vi "Build Swept Freq Vectors.vi"(5 "Low or High (T=Low)":bool=TRUE, 6 "Freq. Increment MHz":dbl=0.001 min=0.001, 7 "Base Order (0)":u8, 8 "Carrier 2":cluster{"Low Freq":dbl, "High Freq":dbl} {"Low Freq" format="%.2f"; "High Freq" format="%.2f"}, 9 "Carrier 1":cluster{"Low Freq":dbl, "High Freq":dbl} {"Low Freq" format="%.2f"; "High Freq" format="%.2f"}, 10 "Rx High Freq":dbl format="%.2f", 11 "Rx Low Freq":dbl format="%.2f") -> (0 "F2>F1 Changeover Index":i32, 1 "F1 RxStep":dbl, 2 "F2 RxStep":dbl, 3 "Freq Sweep":cluster{"F(C1)":dbl, "F(C2)":dbl}[](array[cluster]) {"F(C2)" format="%.6f"; "F(C1)" format="%.6f"})   [LabVIEW 2011]
doc: "Accepts Carrier min, max and Rx Band min, max values along with an increment to generate two 3-D arrays.\n\nThe arrays contain the F1, F2, F(IM), and LO frequencies. The first index of each array selects IM3, 5, 7, and 9. The second index selects the individual frequency vector desired. The third index selects the individual element within each vector.\n\nThe output arrays are arranged so that the IM product appears increasing."
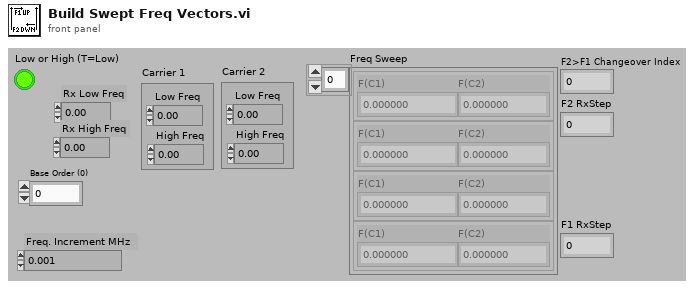
[diagram p1: front panel]
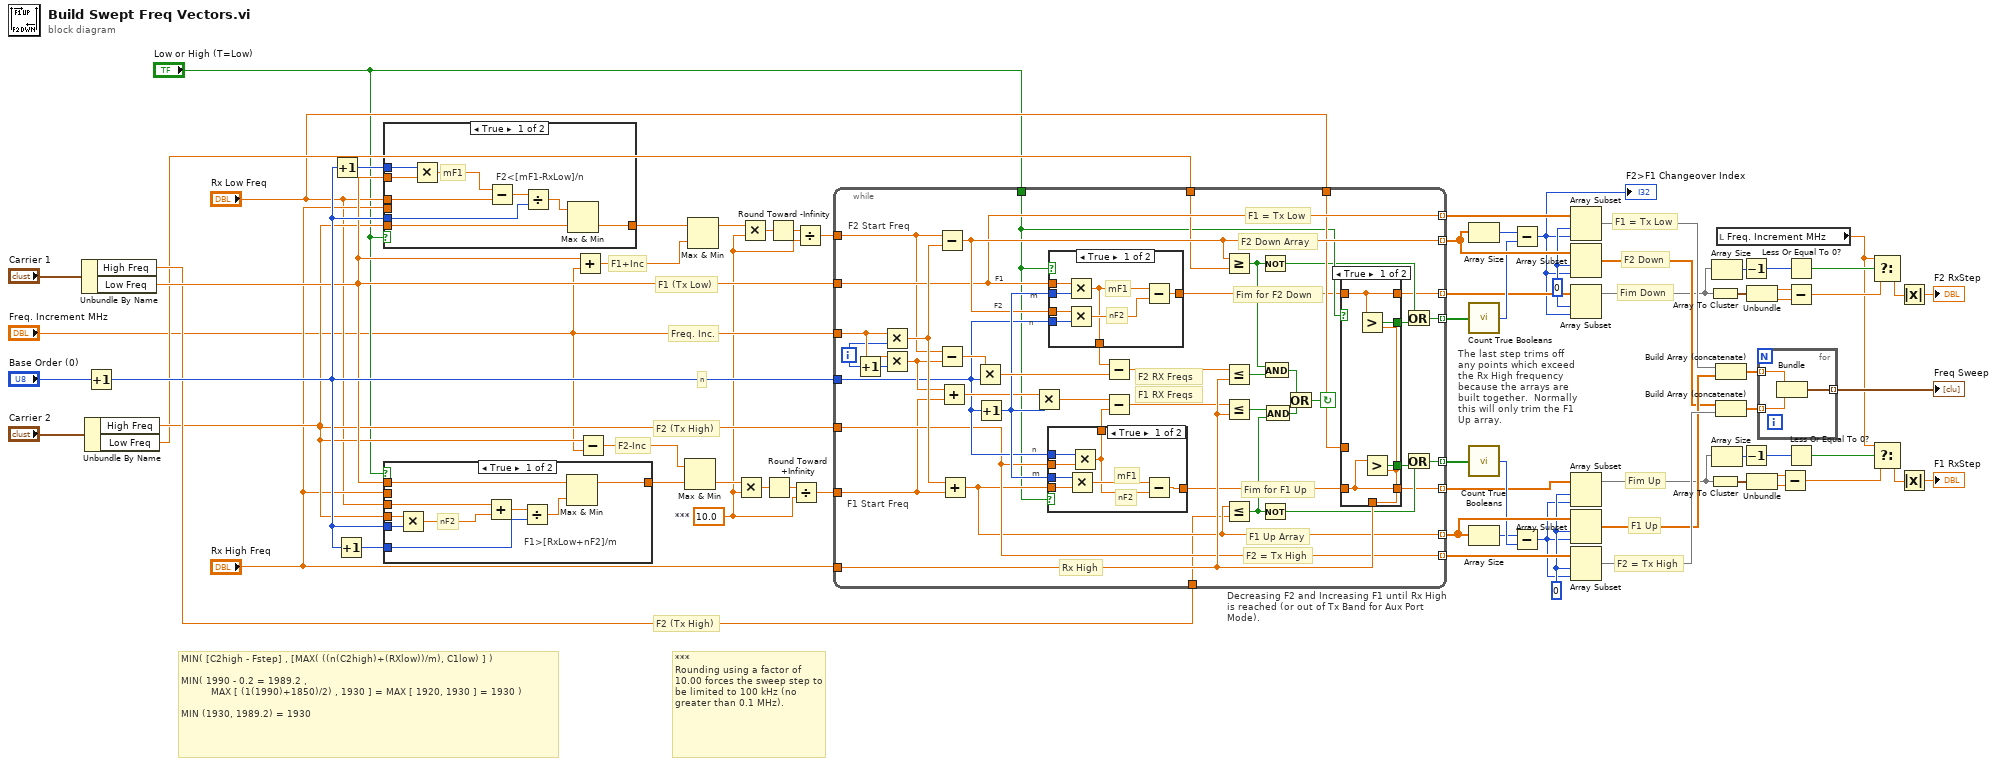
[diagram p0: block diagram]
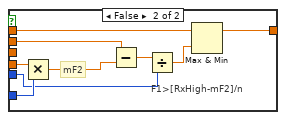
[diagram p2: hidden frame]
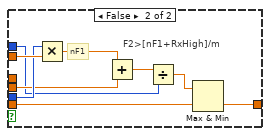
[diagram p3: hidden frame]
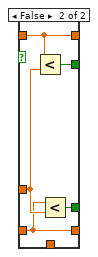
[diagram p4: hidden frame]
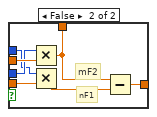
[diagram p5: hidden frame]
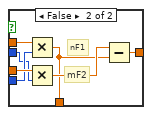
[diagram p6: hidden frame]
diagram:
  w1 = 10.0  # ***
  w31 = 0 ("Array Index")
  w28 = 0 ("Array Index")
  # "*** \nRounding using a factor of 10.00 forces the sweep step to be limited to 100 kHz (no greater than 0.1 MHz)."
  # "F2 (Tx High)"
  # "Fim Up"
  # "Fim Down"
  # "MIN( [C2high - Fstep] , [MAX( ((n(C2high)+(RXlow))/m), C1low) ] )\n\nMIN( 1990 - 0.2 = 1989.2 ,\n          MAX [ (1(1990)+1850)/2) , 1930 ] = MAX [ 1920, 1930 ] = 1930 )\n\nMIN (1930, 1989.2) = 1930"
  # "F2 = Tx High"
  # "F1 Up"
  # "F2 Down"
  # "F1 = Tx Low"
  # "The last step trims off\nany points which exceed\nthe Rx High frequency\nbecause the arrays are\nbuilt together.  Normally\nthis will only trim the F1\nUp array."
  # "F2-Inc"
  # "Freq. Inc."
  # "F2 (Tx High)"
  # "F1+Inc"
  # "n"
  # "F1 (Tx Low)"
  n1 = Unbundle By Name("Carrier 1") -> ("High Freq"=w41:dbl, "Low Freq"=w42:dbl)
  n2 = Unbundle By Name("Carrier 2") -> ("High Freq"=w39:dbl, "Low Freq"=w38:dbl)
  n3 = Increment(x="Base Order (0)") -> (x+1=w70:u8)
  n4 = Increment(x=w70) -> (x+1=w65:u8)
  n5 = Increment(x=w70) -> (x+1=w67:u8)
  n6 = case shown="True" "Low or High (T=Low)" {
    tunnel: "Rx Low Freq" -> [w80 _]
    tunnel: w70 -> [w79 w84]
    tunnel: [w76 w81] -> w68
    tunnel: w65 -> [w74 w82]
    tunnel: w42 -> [w73 w86]
    tunnel: w39 -> [w72 w85]
    tunnel: "Rx High Freq" -> [_ w83]
    frame True {
      # "F2<[mF1-RxLow]/n"
      # "mF1"
      n7 = Multiply(x=w74, y=w73) -> (x*y=w78:dbl)
      n8 = Subtract(x=w78, y=w80) -> (x-y=w77:dbl)
      n9 = Divide(x=w77, y=w79) -> (x/y=w75:dbl)
      n10 = Max & Min(x=w75, y=w72) -> (min(x,y)=w76:dbl)  [unwired: 1 out]
    }
    frame False {
      # "F2>[nF1+RxHigh]/m"
      # "nF1"
      n11 = Multiply(x=w84, y=w86) -> (x*y=w89:dbl)
      n12 = Add(x=w89, y=w83) -> (x+y=w88:dbl)
      n13 = Divide(x=w88, y=w82) -> (x/y=w87:dbl)
      n14 = Max & Min(x=w87, y=w85) -> (min(x,y)=w81:dbl)  [unwired: 1 out]
    }
  }
  n15 = case shown="True" "Low or High (T=Low)" {
    tunnel: "Rx Low Freq" -> [w98 _]
    tunnel: w70 -> [w97 w99]
    tunnel: w67 -> [w95 w101]
    tunnel: [w92 w104] -> w66
    tunnel: w42 -> [w91 w103]
    tunnel: w39 -> [w90 w102]
    tunnel: "Rx High Freq" -> [_ w100]
    frame True {
      # "nF2"
      # "F1>[RxLow+nF2]/m"
      n16 = Multiply(x=w90, y=w97) -> (x*y=w94:dbl)
      n17 = Add(x=w98, y=w94) -> (x+y=w96:dbl)
      n18 = Divide(x=w96, y=w95) -> (x/y=w93:dbl)
      n19 = Max & Min(x=w91, y=w93) -> (max(x,y)=w92:dbl)  [unwired: 1 out]
    }
    frame False {
      # "mF2"
      # "F1>[RxHigh-mF2]/n"
      n20 = Multiply(x=w102, y=w101) -> (x*y=w106:dbl)
      n21 = Subtract(x=w100, y=w106) -> (x-y=w107:dbl)
      n22 = Divide(x=w107, y=w99) -> (x/y=w105:dbl)
      n23 = Max & Min(x=w103, y=w105) -> (max(x,y)=w104:dbl)  [unwired: 1 out]
    }
  }
  n24 = Add(x=w42, y="Freq. Increment MHz") -> (x+y=w69:dbl)
  n25 = Subtract(x=w39, y="Freq. Increment MHz") -> (x-y=w64:dbl)
  n26 = Max & Min(x=w64, y=w66) -> (min(x,y)=w45:dbl)  [unwired: 1 out]
  n27 = Max & Min(x=w68, y=w69) -> (max(x,y)=w47:dbl)  [unwired: 1 out]
  n28 = Multiply(x=w45, y=w1) -> (x*y=w2:dbl)
  n29 = Multiply(x=w47, y=w1) -> (x*y=w5:dbl)
  n30 = Round Toward +Infinity(x=w2) -> (ceil(x): smallest int >= x=w3:dbl)
  n31 = Round Toward -Infinity(1:w5) -> (0:w4:dbl)
  n32 = Divide(x=w3, y=w1) -> (x/y=w44:dbl)
  n33 = Divide(x=w4, y=w1) -> (x/y=w46:dbl)
  n34 = while "Decreasing F2 and Increasing F1 until Rx High is reached (or out of Tx Band for Aux Port Mode)." {
    tunnel: w44 -> [w127]
    tunnel: w46 -> [w128]
    tunnel: [w125] -> w56 mode=indexing
    tunnel: [w126] -> w57 mode=indexing
    tunnel: [w129] -> w62 mode=indexing
    tunnel: [w130] -> w63 mode=indexing
    tunnel: w39 -> [w130]
    tunnel: "Rx High Freq" -> [w136]
    tunnel: w70 -> [w140]
    tunnel: [w132] -> w60 mode=indexing
    tunnel: [w131] -> w61 mode=indexing
    tunnel: "Freq. Increment MHz" -> [w148]
    tunnel: w42 -> [w131]
    tunnel: w38 -> [w121]
    tunnel: w41 -> [w120]
    tunnel: "Rx Low Freq" -> [w119]
    tunnel: "Low or High (T=Low)" -> [w118]
    tunnel: [w109] -> w32 mode=indexing
    tunnel: [w108] -> w29 mode=indexing
    i -> [w147]
    stop <- w137 continue-if-true
    # "F2 RX Freqs"
    # "F1 RX Freqs"
    # "n"
    # "m"
    # "F2"
    # "F1"
    # "n"
    # "m"
    # "F1 Start Freq"
    # "F2 Start Freq"
    # "Rx High"
    # "F1 Up Array"
    # "Fim for F2 Down"
    # "Fim for F1 Up"
    # "F2 = Tx High"
    # "F2 Down Array"
    # "F1 = Tx Low"
    n35 = Increment(x=w147) -> (x+1=w146:i32)
    n36 = Multiply(x=w148, y=w147) -> (x*y=w144:dbl)
    n37 = Multiply(x=w148, y=w146) -> (x*y=w143:dbl)
    n38 = Subtract(x=w128, y=w144) -> (x-y=w132:dbl)
    n39 = Subtract(x=w128, y=w143) -> (x-y=w150:dbl)
    n40 = Add(x=w143, y=w127) -> (x+y=w141:dbl)
    n41 = Add(x=w144, y=w127) -> (x+y=w129:dbl)
    n42 = Multiply(x=w150, y=w140) -> (x*y=w149:dbl)
    n43 = Increment(x=w140) -> (x+1=w142:u8)
    n44 = Multiply(x=w141, y=w142) -> (x*y=w139:dbl)
    n45 = case shown="True" w118 {
      tunnel: w142 -> [w167 w171]
      tunnel: w140 -> [w166 w168]
      tunnel: [w164 w170] -> w138
      tunnel: [w163 w174] -> w110
      tunnel: w130 -> [w162 w173]
      tunnel: w129 -> [w161 w172]
      frame True {
        # "mF1"
        # "nF2"
        n46 = Multiply(x=w167, y=w161) -> (x*y=w165:dbl)
        n47 = Multiply(x=w166, y=w162) -> (x*y=w164:dbl)
        n48 = Subtract(x=w165, y=w164) -> (x-y=w163:dbl)
      }
      frame False {
        # "mF2"
        # "nF1"
        n49 = Multiply(x=w171, y=w173) -> (x*y=w170:dbl)
        n50 = Multiply(x=w168, y=w172) -> (x*y=w169:dbl)
        n51 = Subtract(x=w170, y=w169) -> (x-y=w174:dbl)
      }
    }
    n52 = case shown="True" w118 {
      tunnel: [w180 w182] -> w145
      tunnel: w142 -> [w179 w183]
      tunnel: w140 -> [w178 w184]
      tunnel: w132 -> [w177 w188]
      tunnel: [w176 w187] -> w117
      tunnel: w131 -> [w175 w186]
      frame True {
        # "nF2"
        # "mF1"
        n53 = Multiply(x=w175, y=w179) -> (x*y=w180:dbl)
        n54 = Multiply(x=w177, y=w178) -> (x*y=w181:dbl)
        n55 = Subtract(x=w180, y=w181) -> (x-y=w176:dbl)
      }
      frame False {
        # "mF2"
        # "nF1"
        n56 = Multiply(x=w186, y=w184) -> (x*y=w182:dbl)
        n57 = Multiply(x=w188, y=w183) -> (x*y=w185:dbl)
        n58 = Subtract(x=w185, y=w182) -> (x-y=w187:dbl)
      }
    }
    n59 = Subtract(x=w145, y=w149) -> (x-y=w116:dbl)
    n60 = Subtract(x=w139, y=w138) -> (x-y=w111:dbl)
    n61 = Greater Or Equal?(x=w132, y=w121) -> (x >= y?=w124:bool)
    n62 = Less Or Equal?(x=w116, y=w136) -> (x <= y?=w135:bool)
    n63 = Less Or Equal?(x=w111, y=w136) -> (x <= y?=w112:bool)
    n64 = Less Or Equal?(x=w129, y=w120) -> (x <= y?=w113:bool)
    n65 = Not(x=w124) -> (.not. x?=w115:bool)
    n66 = Not(x=w113) -> (.not. x?=w122:bool)
    n67 = And(x=w124, y=w135) -> (x .and. y?=w134:bool)
    n68 = And(x=w112, y=w113) -> (x .and. y?=w133:bool)
    n69 = Or(x=w134, y=w133) -> (x .or. y?=w137:bool)
    n70 = case shown="True" w118 {
      tunnel: w110 -> [w152 w156]
      tunnel: w136 -> [w153 _]
      tunnel: w117 -> [w151 w157]
      tunnel: [w155 w160] -> w114
      tunnel: [w154 w159] -> w123
      tunnel: w119 -> [_ w158]
      tunnel: [w151 w157] -> w109
      tunnel: [w152 w156] -> w108
      frame True {
        n71 = Greater?(x=w151, y=w153) -> (0:w155:bool)
        n72 = Greater?(x=w152, y=w153) -> (0:w154:bool)
      }
      frame False {
        n73 = Less?(x=w157, y=w158) -> (x < y?=w160:bool)
        n74 = Less?(x=w156, y=w158) -> (x < y?=w159:bool)
      }
    }
    n75 = Or(x=w115, y=w114) -> (x .or. y?=w125:bool)
    n76 = Or(x=w122, y=w123) -> (x .or. y?=w126:bool)
  }
  n77 = Array Size(array=w60) -> (size(s)=w50:i32)
  n78 = call "Count True Booleans.vi"("Boolean Array"=w56) -> ("Number of True"=w55:i32)  [unwired: 4 out]
  n79 = call "Count True Booleans.vi"("Boolean Array"=w57) -> ("Number of True"=w54:i32)  [unwired: 4 out]
  n80 = Array Size(array=w62) -> (size(s)=w51:i32)
  n81 = Subtract(x=w50, y=w55) -> (x-y=w30:i32)
  "F2>F1 Changeover Index" <- w30
  n82 = Subtract(x=w51, y=w54) -> (x-y=w27:i32)
  n83 = Array Subset(array=w61, index=w31, length=w30) -> (w59:dbl[])
  n84 = Array Subset(array=w60, index=w31, length=w30) -> (w33:dbl[])
  n85 = Array Subset(array=w32, index=w31, length=w30) -> (w18:dbl[])
  n86 = Array Subset(array=w29, index=w28, length=w27) -> (w9:dbl[])
  n87 = Array Subset(array=w62, index=w28, length=w27) -> (w49:dbl[])
  n88 = Array Subset(array=w63, index=w28, length=w27) -> (w58:dbl[])
  n89 = Array To Cluster(array=w18) -> (cluster=w22:cluster{"[0]":dbl, "[1]":dbl})
  n90 = Array To Cluster(array=w9) -> (cluster=w26:cluster{"[0]":dbl, "[1]":dbl})
  n91 = Array Size(array=w18) -> (size(s)=w17:i32)
  n92 = Array Size(array=w9) -> (size(s)=w10:i32)
  n93 = Build Array (concatenate)(w59, w49) -> (w53:dbl[])
  n94 = Build Array (concatenate)(w33, w58) -> (w52:dbl[])
  n95 = local read "Freq. Increment MHz"() -> (w7:dbl)
  n96 = Decrement(x=w17) -> (x-1=w16:i32)
  n97 = Decrement(x=w10) -> (x-1=w11:i32)
  n98 = Unbundle(w22) -> ("[0]"=w20:dbl, "[1]"=w19:dbl)
  n99 = Unbundle(w26) -> ("[0]"=w24:dbl, "[1]"=w23:dbl)
  n100 = for {
    tunnel: w53 -> [w191] mode=indexing
    tunnel: w52 -> [w190] mode=indexing
    tunnel: [w189] -> w48 mode=indexing
    n101 = Bundle("Low Freq"=w191, "High Freq"=w190) -> (w189:cluster{"Low Freq":dbl, "High Freq":dbl})  [unwired: 1 out]
  }
  "Freq Sweep" <- w48
  n102 = Subtract(x=w24, y=w23) -> (x-y=w8:dbl)
  n103 = Less Or Equal To 0?(x=w16) -> (x <= 0?=w15:bool)
  n104 = Subtract(x=w20, y=w19) -> (x-y=w14:dbl)
  n105 = Less Or Equal To 0?(x=w11) -> (x <= 0?=w12:bool)
  n106 = Select(t=w7, s=w15, f=w14) -> (s? t:f=w13:dbl)
  n107 = Select(t=w7, s=w12, f=w8) -> (s? t:f=w6:dbl)
  n108 = Absolute Value(x=w13) -> (abs(x)=→"F2 RxStep":dbl)
  n109 = Absolute Value(x=w6) -> (abs(x)=→"F1 RxStep":dbl)
